vi "Usage2.vi"() -> ()   [LabVIEW 2017]
uses:
  Tests/Support/Consumers/Test UI Consumer/Test UI Consumer.lvclass
  C:/github/niveristand-custom-device-message-library/Source/Consumer/Abstract Consumer/Abstract Consumer.lvclass
  Producer/Abstract Producer/Abstract Producer.lvclass
  Message Queue/Message Queue/Message Queue.lvclass
  C:/github/niveristand-custom-device-message-library/Source/Message Queue/Abstract Message Queue/Abstract Message Queue.lvclass
  Parameters/Abstract Init Parameters/Abstract Init Parameters.lvclass
  Message/Shutdown Message/Shutdown Message.lvclass
  C:/github/niveristand-custom-device-message-library/Source/Message/Abstract Message/Abstract Message.lvclass
  Tests/Support/Messages/Test UI Message/Test UI Message.lvclass
  Consumer/Abstract Consumer/Abstract Consumer.lvclass
panel:
  in  "Test":bool
  in  "stop":bool
  out "error out":errorcluster
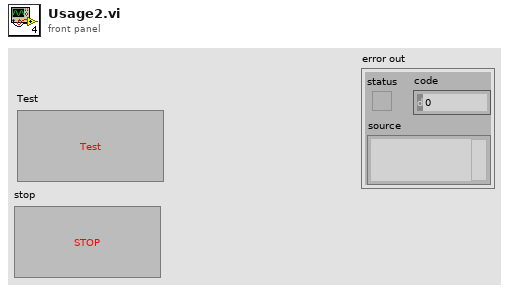
[diagram p1: front panel]
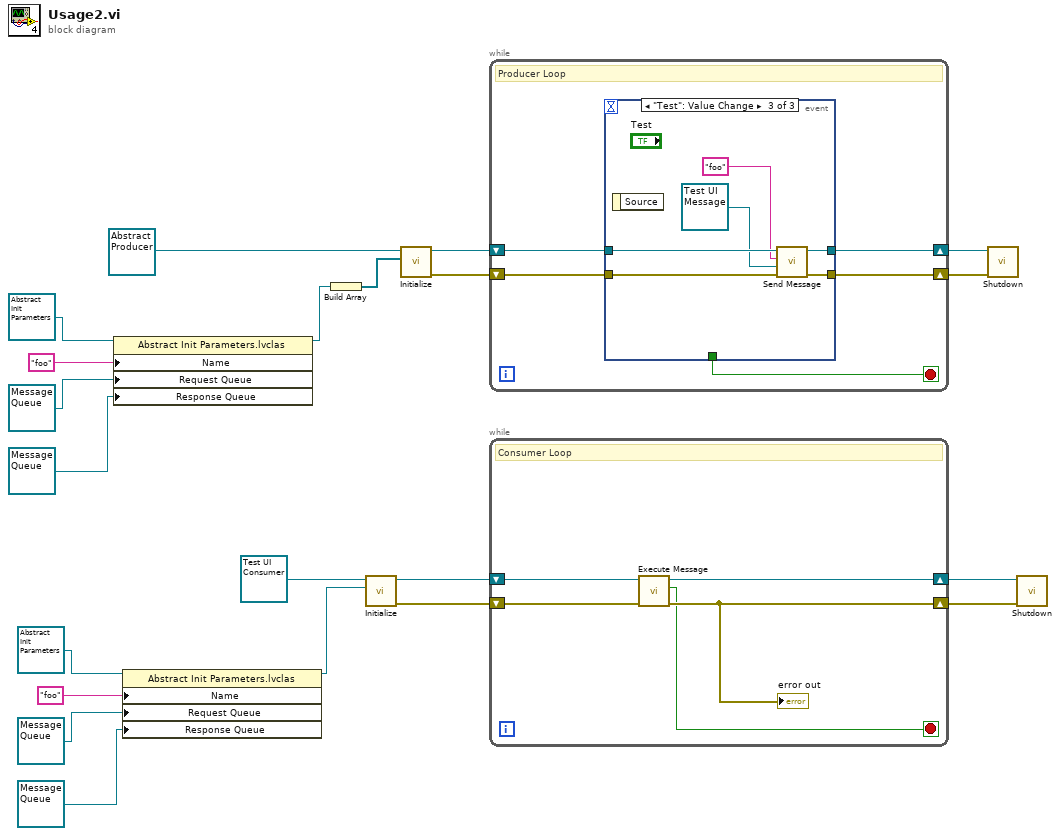
[diagram p0: block diagram]
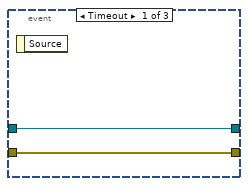
[diagram p2: hidden frame]
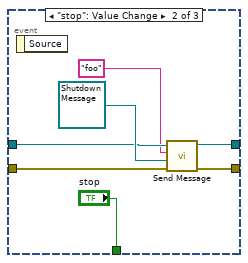
[diagram p3: hidden frame]
diagram:
  n1 = property class="Abstract Init Parameters.lvclas"(reference=refnum<class "Abstract Init Parameters.lvclass"> refnum ("Message Queue Library.lvlib:Abstract Init Parameters.lvclass"), "Name"="foo", "Request Queue"=refnum<class "Message Queue.lvclass"> refnum ("Message Queue Library.lvlib:Message Queue.lvclass"), "Response Queue"=refnum<class "Message Queue.lvclass"> refnum ("Message Queue Library.lvlib:Message Queue.lvclass")) -> (reference out=w6:refnum<class "Abstract Init Parameters.lvclass">)  [unwired: 1 in, 1 out]
  n2 = property class="Abstract Init Parameters.lvclas"(reference=refnum<class "Abstract Init Parameters.lvclass"> refnum ("Message Queue Library.lvlib:Abstract Init Parameters.lvclass"), "Name"="foo", "Request Queue"=refnum<class "Message Queue.lvclass"> refnum ("Message Queue Library.lvlib:Message Queue.lvclass"), "Response Queue"=refnum<class "Message Queue.lvclass"> refnum ("Message Queue Library.lvlib:Message Queue.lvclass")) -> (reference out=w12:refnum<class "Abstract Init Parameters.lvclass">)  [unwired: 1 in, 1 out]
  n3 = Build Array(w6) -> (w13:refnum<class "Abstract Init Parameters.lvclass">[])
  n4 = call "Initialize.vi"("Parameters in"=w12, "Abstract Consumer in"=refnum<class "Test UI Consumer.lvclass"> refnum ("Message Queue Library.lvlib:Test Consumer.lvclass")) -> ("error out"=w19:errorcluster, "Abstract Consumer out"=w20:refnum<class "Test UI Consumer.lvclass">)  [unwired: 8 in]
  n5 = call "Initialize.vi"("Parameters in"=w13, "Abstract Producer in"=refnum<class "Abstract Producer.lvclass"> refnum ("Message Queue Library.lvlib:Abstract Producer.lvclass")) -> ("error out"=w2:errorcluster, "Abstract Producer out"=w11:refnum<class "Abstract Producer.lvclass">)  [unwired: 8 in]
  n6 = while {
    shift-right: [w24] -> w5
    shift-left: w11 -> [w25]
    shift-right: [w22] -> w1
    shift-left: w2 -> [w23]
    stop <- w26 stop-if-true
    # "Producer Loop"
    n7 = event shown="[2] \"Test\": Value Change" {
      selector: _ -> [_ _ _]
      dyn-events: _ -> [_ _ _]
      timeout: _ -> [_ _ _]
      tunnel: [_ "stop" _] -> w26
      tunnel: w25 -> [w28 w33 w41]
      tunnel: [w28 w32 w40] -> w24
      tunnel: w23 -> [w27 w30 w37]
      tunnel: [w27 w29 w36] -> w22
      event Timeout {
        n8 = event-data() -> ()  [unwired: 1 in, 1 out]
      }
      event "stop": Value Change {
        n9 = event-data() -> ()  [unwired: 1 in, 1 out]
        n10 = call-dynamic "Send Message.vi"("error in (no error)"=w30, "Message in"=refnum<class "Shutdown Message.lvclass"> refnum ("Message Queue Library.lvlib:Shutdown Message.lvclass"), "Consumer in"="foo", "Abstract Producer in"=w33) -> ("error out"=w29:errorcluster, "Abstract Producer out"=w32:refnum<class "Abstract Producer.lvclass">)  [unwired: 5 in, 1 out]
      }
      event "Test": Value Change {
        n11 = event-data() -> ()  [unwired: 1 in, 1 out]
        n12 = call-dynamic "Send Message.vi"("error in (no error)"=w37, "Message in"=refnum<class "Test UI Message.lvclass"> refnum ("Message Queue Library.lvlib:Test Message.lvclass"), "Consumer in"="foo", "Abstract Producer in"=w41) -> ("error out"=w36:errorcluster, "Abstract Producer out"=w40:refnum<class "Abstract Producer.lvclass">)  [unwired: 5 in, 1 out]
      }
    }
  }
  n13 = while {
    shift-right: [w45] -> w4
    shift-left: w20 -> [w46]
    shift-right: [w43] -> w3
    shift-left: w19 -> [w44]
    stop <- w42 stop-if-true
    # "Consumer Loop"
    n14 = call "Execute Message.vi"("error in (no error)"=w44, "Abstract Consumer in"=w46) -> ("error out"=w43:errorcluster, "Stop?"=w42:bool, "Abstract Consumer out"=w45:refnum<class "Abstract Consumer.lvclass">)  [unwired: 7 in]
    "error out" <- w43
  }
  n15 = call "Shutdown.vi"("error in (no error)"=w1, "Abstract Producer in"=w5) -> ()  [unwired: 8 in, 2 out]
  n16 = call "Shutdown.vi"("error in (no error)"=w3, "Abstract Consumer in"=w4) -> ()  [unwired: 8 in, 2 out]
